vi "Targets File Work Around.vi"(8 "error in (no error)":errorcluster, 11 "overrides file in":path=path "Assets/DummyProperty.ini") -> (0 "error out":errorcluster, 3 "overrides file out":path=path "Assets/DummyProperty.ini")   [LabVIEW 2027, in "VeriStandTestCaseSystemTests.lvclass"]
uses:
  VeriStandTestCaseSystemTests.lvclass
  <vilib>/Utility/config.llb/Write Key (String).vi
  Source/VeriStandTestUtilities/VeriStandTestUtilities.lvlib
  <vilib>/Utility/config.llb/NI_LVConfig.lvlib
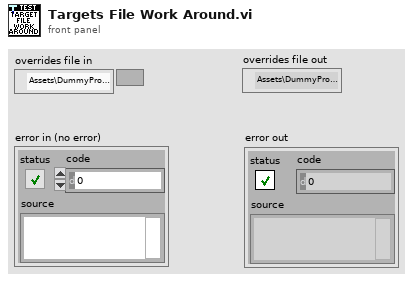
[diagram p1: front panel]
types:
  T1 = typedef "VeriStandTestUtilities.lvlib/TargetsConfiguration.ctl" = cluster{"Supported Targets":cluster{"IP Address / Hostname":string, "Target Platform":T2}[], "Active Configuration":T2}
  T2 = typedef "VeriStandTestUtilities.lvlib/TargetPlatform.ctl" = enum16{"Windows", "Linux64CRIO", "Linux64PXI", "LinuxARM", "PharLap"}
  T3 = cluster{"IP Address / Hostname":string, "Target Platform":T2}[]
  T4 = typedef "NI_LVConfig.lvlib/Config Data RefNum.ctl" = refnum<k1>
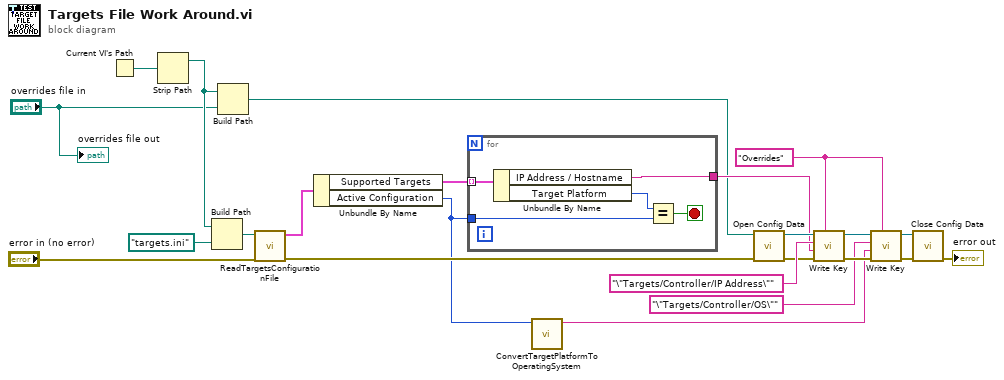
[diagram p0: block diagram]
diagram:
  w5 = "Overrides" ("section")
  n1 = Current VI's Path() -> (path=w23:path)
  n2 = Strip Path(path=w23) -> (stripped path=w21:path)  [unwired: 1 out]
  n3 = Build Path(base path=w21, name or relative path=path "targets.ini" ("overrides files")) -> (appended path=w20:path)
  n4 = Build Path(base path=w21, name or relative path="overrides file in") -> (appended path=w11:path)
  n5 = call "ReadTargetsConfigurationFile.vi"("error in (no error)"="error in (no error)", "targets.ini file"=w20) -> ("error out"=w16:errorcluster, "Targets Configuration"=w18:T1)  [unwired: 8 in]
  n6 = Unbundle By Name(w18) -> ("Supported Targets"=w17:T3, "Active Configuration"=w3:T2)
  n7 = for {
    tunnel: w17 -> [w28] mode=indexing
    tunnel: w3 -> [w26]
    tunnel: [w24] -> w12
    stop <- w25 stop-if-true
    n8 = Unbundle By Name(w28) -> ("IP Address / Hostname"=w24:string, "Target Platform"=w27:T2)
    n9 = Equal?(x=w27, y=w26) -> (x = y?=w25:bool)
  }
  n10 = call "ConvertTargetPlatformToOperatingSystem.vi"("Platform"=w3) -> ("Operating System"=w2:string)  [unwired: 10 in]
  n11 = call <vilib>:"Open Config Data.vi"("error in (no error)"=w16, "configuration file path"=w11) -> ("error out"=w13:errorcluster, "refnum"=w15:T4)  [unwired: 7 in, 1 out]
  n12 = call-poly <vilib>:"Write Key.vi"("section"=w5, "error in (no error)"=w13, "value"=w12, "key"="\"Targets/Controller/IP Address\"", "refnum"=w15) -> ("error out"=w9:errorcluster, "refnum out"=w8:T4)  [unwired: 4 in, 1 out]
  n13 = call-poly <vilib>:"Write Key.vi"("section"=w5, "error in (no error)"=w9, "value"=w2, "key"="\"Targets/Controller/OS\"", "refnum"=w8) -> ("error out"=w6:errorcluster, "refnum out"=w7:T4)  [unwired: 4 in, 1 out]
  n14 = call <vilib>:"Close Config Data.vi"("error in (no error)"=w6, "refnum"=w7) -> ("error out"=→"error out":errorcluster)  [unwired: 8 in, 1 out]
  "overrides file out" <- "overrides file in"
